vi "TurnArc.vi"(10 "angle":dbl, 11 "radius":dbl) -> ()   [LabVIEW 2019]
uses:
  <vilib>/Rock Robotics/WPI/Utilities/WPI_GetSetVariantRefNum.vi
  <vilib>/Rock Robotics/WPI/RobotDrive/WPI_RobotDriveArcadeDrive_Standard(NoSaturation).vi
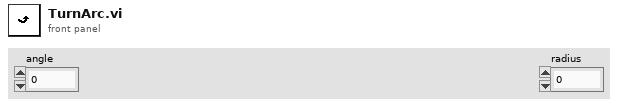
[diagram p1: front panel]
types:
  T1 = typedef "WPI_EncoderDevRef.ctl" = cluster{"DevStatus":errorcluster, "EncoderIndex":T2, "CounterIndex":T3, "DistancePerCount":dbl, "Decoding Type":T4}
  T2 = typedef "FPGA_EncoderIdx.ctl" = enum8{"Enc 0", "Enc 1", "Enc 2", "Enc 3", "Enc 4", "Enc 5", "Enc 6", "Enc 7", "Invalid"}
  T3 = typedef "FPGA_CounterCtrSystemIndex.ctl" = enum8{"Ctr 0", "Ctr 1", "Ctr 2", "Ctr 3", "Ctr 4", "Ctr 5", "Ctr 6", "Ctr 7", "Invalid"}
  T4 = typedef "WPI_EncoderType.ctl" = enum16{"1x", "2x", "4x"}
  T5 = typedef "WPI_RobotDriveDevRef.ctl" = cluster{"DevStatus":errorcluster, "Motors[]":T6[], "Square Inputs":bool, "Max Output":dbl}
  T6 = typedef "WPI_MotorControlDeviceRef.ctl" = cluster{"DeviceStatus":errorcluster, "Type":T7, "PWM":cluster{"PWM Channel":T8, "DeadBand":T9}, "CAN":cluster{"Device Number":u8, "SetOutput VI Ref":variant, "GetOutput VI Ref":variant, "Enable VI Ref":variant, "Disable VI Ref":variant, "Data":variant}, "Invert":bool, "DIO PWM":cluster{"PWM \"Enable\" Channel":T8, "DIOChannel":T10, "PWM Rate":dbl}}
  T7 = typedef "WPI_MotorControlType.ctl" = enum16{"PWM", "CAN", "DIO PWM"}
  T8 = typedef "FPGA_DIOPWMChannel.ctl" = enum8{"PWM 0", "PWM 1", "PWM 2", "PWM 3", "PWM 4", "PWM 5", "PWM 6", "PWM 7", "PWM 8", "PWM 9", "PWM MXP 0", "PWM MXP 1", "PWM MXP 2", "PWM MXP 3", "PWM MXP 4", "PWM MXP 5", "PWM MXP 6", "PWM MXP 7", "PWM MXP 8", "PWM MXP 9", "Invalid"}
  T9 = typedef "WPI_PWMDeadband.ctl" = cluster{"Name":string, "maxPositivePwm":i32, "minPositivePwm":i32, "centerPwm":i32, "maxNegativePwm":i32, "minNegativePwm":i32, "angularRange":u16}
  T10 = typedef "FPGA_DIOChannel.ctl" = enum8{"DIO 0", "DIO 1", "DIO 2", "DIO 3", "DIO 4", "DIO 5", "DIO 6", "DIO 7", "DIO 8", "DIO 9", "DIO MXP 0", "DIO MXP 1", "DIO MXP 2", "DIO MXP 3", "DIO MXP 4", "DIO MXP 5", "DIO MXP 6", "DIO MXP 7", "DIO MXP 8", "DIO MXP 9", "DIO MXP 10", "DIO MXP 11", "DIO MXP 12", "DIO MXP 13", "DIO MXP 14", "DIO MXP 15", "SPI Port CS1", "SPI Port CS2", "SPI Port CS3", "SPI Port MISO", "SPI Port MOSI", "Invalid"}
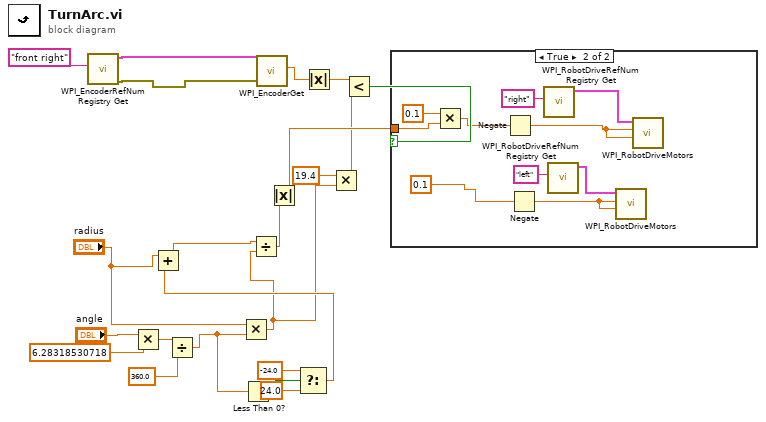
[diagram p0: block diagram]
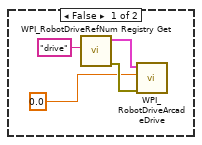
[diagram p2: hidden frame]
diagram:
  n1 = call <vilib>:"WPI_EncoderRefNum Registry Get.vi"("refnum name"="front right") -> ("error out"=w2:errorcluster, "EncoderDevRef"=w1:T1)  [unwired: 9 in]
  n2 = Multiply(x="angle", y=6.28318530718) -> (x*y=w18:dbl)
  n3 = Divide(x=w18, y=360.0) -> (x/y=w16:dbl)
  n4 = Multiply(x="radius", y=w16) -> (x*y=w8:dbl)
  n5 = Less Than 0?(x=w16) -> (x < 0?=w15:bool)
  n6 = call <vilib>:"WPI_EncoderGet.vi"("error in (no error)"=w2, "EncoderDevRef"=w1) -> ("Distance"=w9:dbl)  [unwired: 4 in, 5 out]
  n7 = Select(t=-24.0, s=w15, f=24.0) -> (s? t:f=w11:dbl)
  n8 = Add(x="radius", y=w11) -> (x+y=w10:dbl)
  n9 = Divide(x=w10, y=w8) -> (x/y=w6:dbl)
  n10 = Absolute Value(x=w6) -> (abs(x)=w5:dbl)
  n11 = Absolute Value(x=w9) -> (abs(x)=w21:dbl)
  n12 = Multiply(x=19.4, y=w8) -> (x*y=w4:dbl)
  n13 = Less?(x=w21, y=w4) -> (x < y?=w7:bool)
  n14 = case shown="True" w7 {
    tunnel: w5 -> [_ w31]
    frame False {
      n15 = call <vilib>:"WPI_RobotDriveRefNum Registry Get.vi"("refnum name"="drive") -> ("error out"=w26:errorcluster, "RobotDriveDevRef"=w25:T5)  [unwired: 9 in]
      n16 = call-poly <vilib>:"WPI_RobotDriveArcadeDrive.vi"("error in (no error)"=w26, "X axis value"=0.0, "RobotDriveDevRef"=w25) -> ()  [unwired: 6 in, 3 out]
    }
    frame True {
      n17 = Multiply(x=0.1, y=w31) -> (x*y=w34:dbl)
      n18 = Negate(x=w34) -> (-x=w29:dbl)
      n19 = Negate(x=0.1) -> (-x=w27:dbl)
      n20 = call <vilib>:"WPI_RobotDriveRefNum Registry Get.vi"("refnum name"="right") -> ("RobotDriveDevRef"=w30:T5)  [unwired: 9 in, 1 out]
      n21 = call <vilib>:"WPI_RobotDriveRefNum Registry Get.vi"("refnum name"="left") -> ("RobotDriveDevRef"=w28:T5)  [unwired: 9 in, 1 out]
      n22 = call <vilib>:"WPI_RobotDriveMotors.vi"("RightSpeed"=w27, "LeftSpeed"=w27, "RobotDriveDevRef"=w28) -> ()  [unwired: 6 in, 3 out]
      n23 = call <vilib>:"WPI_RobotDriveMotors.vi"("RightSpeed"=w29, "LeftSpeed"=w29, "RobotDriveDevRef"=w30) -> ()  [unwired: 6 in, 3 out]
    }
  }
